vi "Seconds to Time Unit and Value.vi"(11 "time, s":dbl) -> (3 "time unit and value":cluster{"unit":u16, "value":u16} {"unit" items=["ns", "us", "ms", "s", "m", "h"]})   [LabVIEW 2015, in "PL SOL Instruments Camera.lvclass"]
doc: "Converts <b>time, s</b> to <b>time unit and value</b>."
uses:
  PL SOL Instruments Camera.lvclass
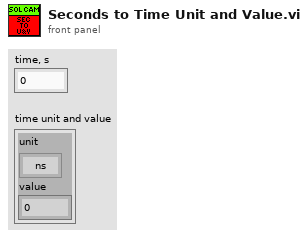
[diagram p1: front panel]
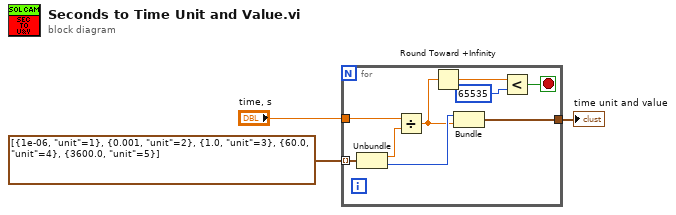
[diagram p0: block diagram]
diagram:
  n1 = for {
    tunnel: "time, s" -> [w12]
    tunnel: cluster{dbl, "unit":u16}[] [{1e-06, "unit"=1}, {0.001, "unit"=2}, {1.0, "unit"=3}, {60.0, "unit"=4}, {3600.0, "unit"=5}] -> [w11] mode=indexing
    tunnel: [w9] -> w1
    stop <- w6 stop-if-true
    n2 = Unbundle(w11) -> (w10:dbl, "unit"=w5:u16)
    n3 = Divide(x=w12, y=w10) -> (x/y=w4:dbl)
    n4 = Round Toward +Infinity(x=w4) -> (ceil(x): smallest int >= x=w8:dbl)
    n5 = Bundle("unit"=w5, w4) -> (w9:cluster{"unit":u16, dbl})  [unwired: 1 in]
    n6 = Less?(x=w8, y=u16 65535 ("value")) -> (x < y?=w6:bool)
  }
  "time unit and value" <- w1
